vi "cDAQ AI Read.vi"(10 "Channel to Cal":T1) -> (0 "Lost Connection":bool, 2 "Available?":bool, 3 "Data":dbl format="%0.2f")   [LabVIEW 2013]
uses:
  Type Defs/cDAQ Type Def (cDAQ).ctl
  Type Defs/TCP Data Stream Mode (PC).ctl
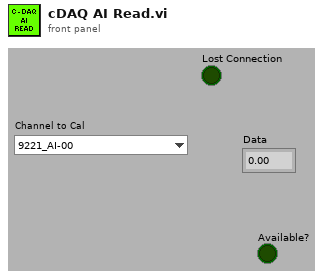
[diagram p1: front panel]
types:
  T1 = typedef "cDAQ Type Def (cDAQ).ctl" = enum16{"9221_AI-00", "9221_AI-01", "9221_AI-02", "9221_AI-03", "9221_AI-04", "9221_AI-05", "9221_AI-06", "9221_AI-07", "9205_AI-00", "9205_AI-01", "9205_AI-02", "9205_AI-03", "9205_AI-04", "9205_AI-05", "9205_AI-06", "9205_AI-07", "9208_AI-00", "9208_AI-01", "9208_AI-02", "9208_AI-03", "9208_AI-04", "9208_AI-05", "9208_AI-06", "9208_AI-07", "9211_TC-00", "9211_TC-01", "9211_TC-02", "9211_TC-03"}
  T2 = typedef "TCP Data Stream Mode (PC).ctl" = enum16{"Init", "Read Data", "Close"}
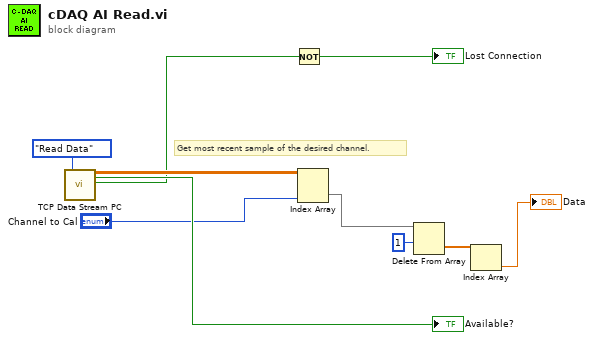
[diagram p0: block diagram]
diagram:
  # "Get most recent sample of the desired channel."
  n1 = call "TCP Data Stream PC.vi"("Mode"=TCP_Data_Stream_Mode_(PC)."Read Data") -> ("Data OUT"=w8:dbl[][], "New Data?"=→"Available?":bool, "Connected?"=w7:bool)  [unwired: 15 in, 1 out]
  n2 = Not(x=w7) -> (.not. x?=→"Lost Connection":bool)
  n3 = Index Array(array=w8, index (col)="Channel to Cal") -> (element=w3:dbl[])  [unwired: 1 in]
  n4 = Delete From Array(array=w3, length=1) -> (deleted portion=w5:dbl[])  [unwired: 1 in, 1 out]
  n5 = Index Array(array=w5) -> (element=→"Data":dbl)  [unwired: 1 in]
